vi "Update.vi"(8 "error in (no error)":errorcluster, 11 "Object":refnum<class "Singleton.lvclass">) -> (0 "error out":errorcluster, 3 "Object (dup)":refnum<class "Singleton.lvclass">, 4 "created new?":bool)   [LabVIEW 2014, in "Singleton.lvlib" / "Singleton.lvclass"]
uses:
  Singleton.lvclass
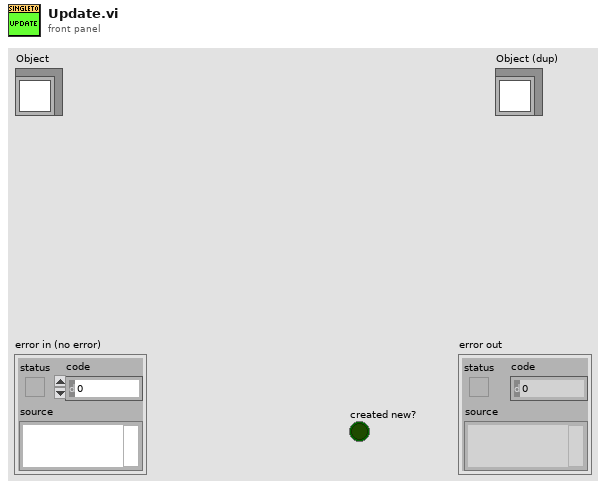
[diagram p1: front panel]
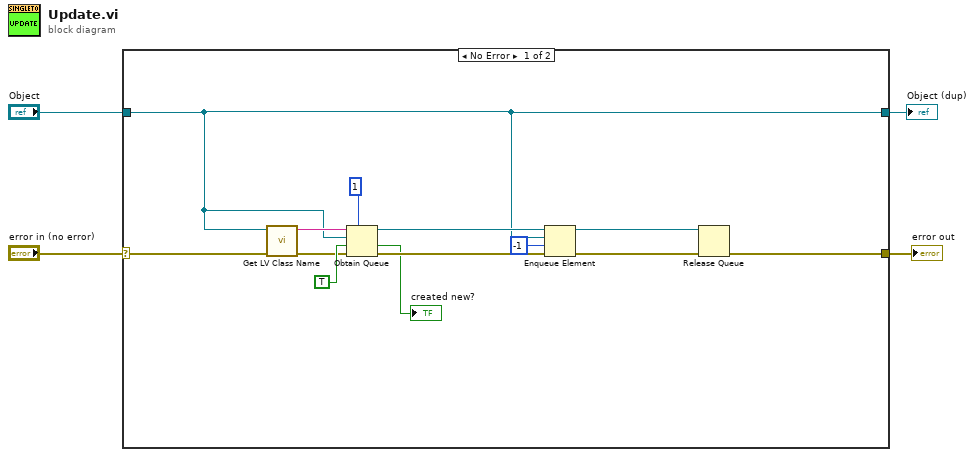
[diagram p0: block diagram]
diagram:
  n1 = case shown="No Error" "error in (no error)" {
    selector: "error in (no error)" -> [w14 w19]
    tunnel: [w7 w19] -> w3
    tunnel: "Object" -> [w10 w18]
    tunnel: [w10 w18] -> w1
    frame No Error {
      n2 = call <vilib>:"Get LV Class Name.vi"("error in (no error)"=w14, "object"=w10) -> ("error out"=w13:errorcluster, "class name"=w17:string)  [unwired: 8 in]
      n3 = Obtain Queue(max queue size (-1, unlimited)=1, name (unnamed)=w17, element data type=w10, create if not found? (T)=TRUE, error in (no error)=w13) -> (queue out=w12:refnum<queue>, created new?=→"created new?":bool, error out=w11:errorcluster)
      n4 = Enqueue Element(queue=w12, element=w10, timeout in ms (-1)=-1, error in (no error)=w11) -> (queue out=w8:refnum<queue>, error out=w9:errorcluster)  [unwired: 1 out]
      n5 = Release Queue(queue=w8, error in (no error)=w9) -> (error out=w7:errorcluster)  [unwired: 1 in, 2 out]
    }
    frame Error {
    }
  }
  "error out" <- w3
  "Object (dup)" <- w1
